vi "Read_and_Save_Card.vi"(8 "error in (no error)":errorcluster, 10 "index":i32, 11 "Current Image Array":i32[](array[numeric])) -> (0 "error out":errorcluster, 2 "Image Value":i32, 3 "Output Image Array":i32[](array[numeric]))   [LabVIEW 2018]
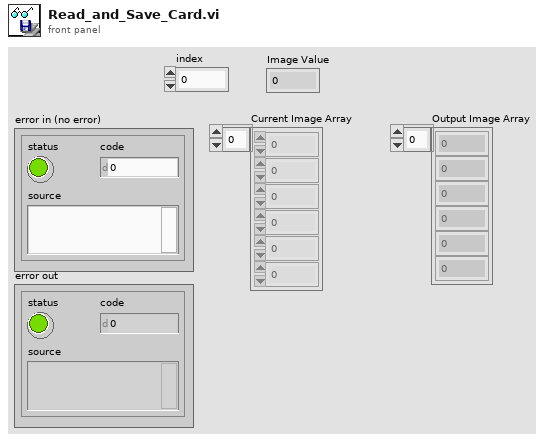
[diagram p1: front panel]
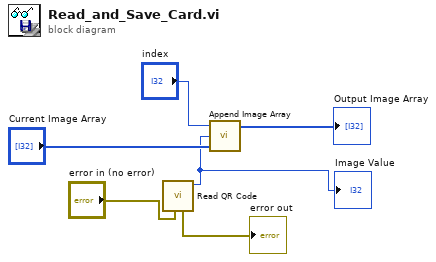
[diagram p0: block diagram]
diagram:
  n1 = call "Read QR Code.vi"("error in (no error)"="error in (no error)") -> ("Image Value"=w3:i32, "error out"=→"error out":errorcluster)  [unwired: 9 in]
  "Image Value" <- w3
  n2 = call "Append Image Array.vi"("index"="index", "New Image Value"=w3, "Current Image Array"="Current Image Array") -> ("Output Image Array"=→"Output Image Array":i32[])  [unwired: 3 in]
